vi "Sequence Execution.vi"() -> ()   [LabVIEW 2013, in "Simple Sequence Editor.lvlib"]
uses:
  Simple Sequence Editor.lvlib
  Types/Execute.PreviewMode.ctl
  Types/Execuction.StateVariables.ctl
  <vilib>/NI Veristand/Execution/Workspace/SystemStateRegEventRef.ctl
  <vilib>/NI Veristand/Execution/Workspace/SystemStateEventRef.ctl
  <vilib>/NI Veristand/Execution/Workspace/WorkspaceAPI.ctl
  Program Files/National Instruments/LabVIEW 2013/examples/NI Veristand/API/Execution API/Sequences/Stimulus Profile Control Tool/Project Execution State.ctl
  NationalInstruments.VeriStand.RealTimeSequenceDefinitionApi
  <vilib>/NI Veristand/Execution/Workspace/NI VeriStand - Get Single Channel Value.vi
  <vilib>/NI Veristand/Execution/Workspace/NI VeriStand - Set Single Channel Value.vi
  <vilib>/NI Veristand/Execution/Workspace/NI_VS Workspace ExecutionAPI.lvlib
  NationalInstruments.VeriStand.ClientAPI
panel:
  out "Current Step":u32
  out "Current Iteration":u32
  in  "NIVS.Project File Path":path
  in  "NIVS.Gateway IP Address":string="localhost"
  in  "NIVS.Workspace Event":refnum<event-registration>
  in  "Preview Mode":T1=enum."Table"
  in  "Start Step":u32 min=1 max=5
  in  "Start Iteration":u32=1 min=1 max=2
  in  "Log Channels":T2(ring)
  in  "Path":path
  in  "Enable Logging":bool
  in  "Abort":bool
  in  "Pause":bool
  in  "Start":bool
  in  "Profiles":string(combo)
  out "Graph":waveform(dbl)[](graph)
  out "Sequence":i32[](listbox)
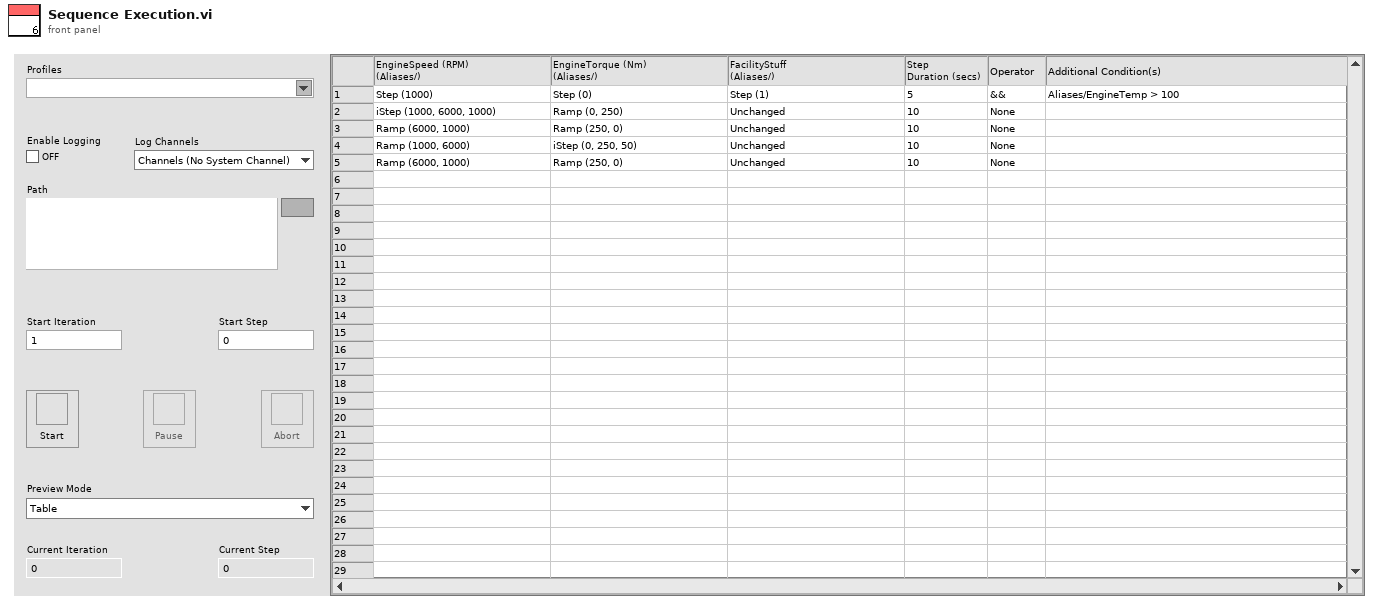
[diagram p1: front panel]
types:
  T1 = typedef "Simple Sequence Editor.lvlib/Execute.PreviewMode.ctl" = enum8{"Graph", "Table"}
  T2 = enum16{"Channels (No System Channel)", "Aliases", "All"}
  T3 = typedef "Simple Sequence Editor.lvlib/Execuction.StateVariables.ctl" = cluster{"Abort":refnum<vi>, "Pause":refnum<vi>, "Enable Logging":refnum<vi>, "Start":refnum<vi>, "Log Channels":refnum<vi>, "Start Iteration":refnum<vi>, "Start Step":refnum<vi>, "Sequence":refnum<vi>, "Preview Mode":refnum<vi>, "Graph":refnum<vi>, "Path":refnum<vi>, "NIVS.Events":cluster{"SequenceRef":refnum<event-registration>, "SystemChangeEventRef":T4, "NIVS.WorkspaceEvents":refnum<event-registration>}, "NIVS.SystemStateRefs":T5, "NIVS.WorkspaceManager":T6, "Abort 2":string, "Step":string, "Iterations":u32, "Iteration":string, "UI.Sequence#ofColumns":i32, "Connected":bool, "Profiles":refnum<vi>, "Events.State":refnum<user-event>, "Events.Test Result":refnum<user-event>, "Events.Progress":refnum<user-event>, "Profile.Ref":refnum<k24>, "Profile.Callback":refnum<k27>, "State":T7, "NIVS.Gateway IP Address":string, "NIVS.Project File Path":path, "Current Step":refnum<vi>, "Current Iteration":refnum<vi>}
  T4 = typedef "NI_VS Workspace ExecutionAPI.lvlib/SystemStateRegEventRef.ctl" = refnum<event-registration>
  T5 = typedef "NI_VS Workspace ExecutionAPI.lvlib/SystemStateEventRef.ctl" = cluster{"CustDatRef":refnum<user-event>, "EvtRef":refnum<k27>}
  T6 = typedef "NI_VS Workspace ExecutionAPI.lvlib/WorkspaceAPI.ctl" = refnum<k24>
  T7 = typedef "Project Execution State.ctl" = enum16{"Idle", "Initializing", "Running", "Paused", "Finalizing", "Complete"}
  T8 = cluster{"Event Registration Refnum":refnum<event-registration>, "SystemChangeEventRef":T4, "NIVS.Workspace Event":refnum<event-registration>}
  T9 = enum8{"Enabled", "Disabled", "Disabled and Grayed Out"}
  T10 = cluster{"SequenceRef":refnum<event-registration>, "SystemChangeEventRef":T4, "NIVS.WorkspaceEvents":refnum<event-registration>}
  T11 = typedef "NI_VS Workspace ExecutionAPI.lvlib/SystemState.ctl" = u8
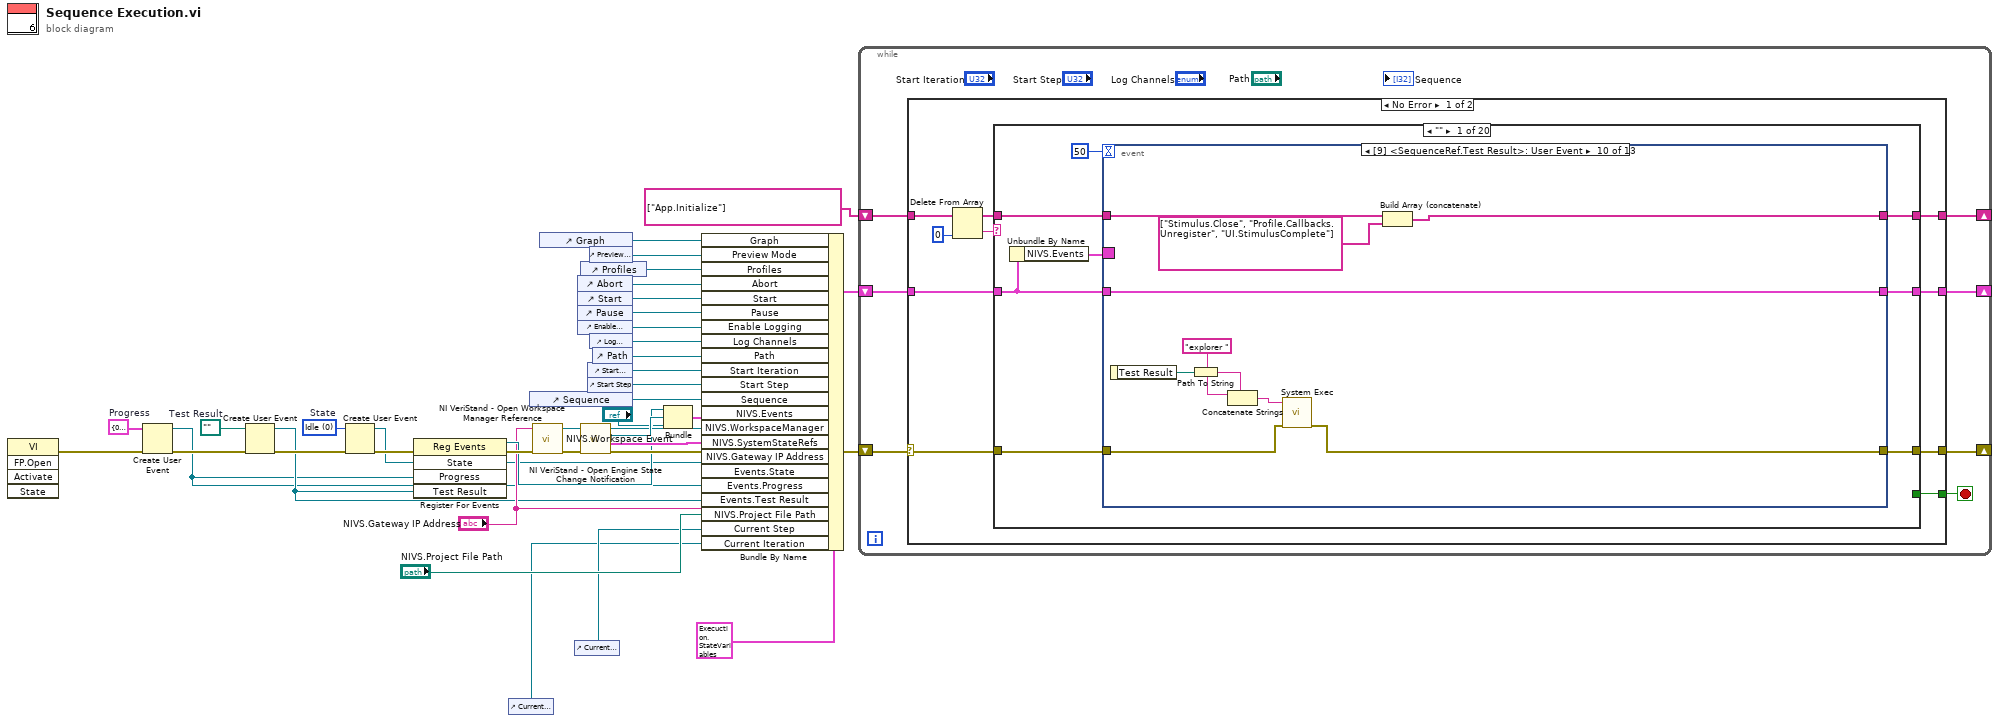
[diagram p0: block diagram]
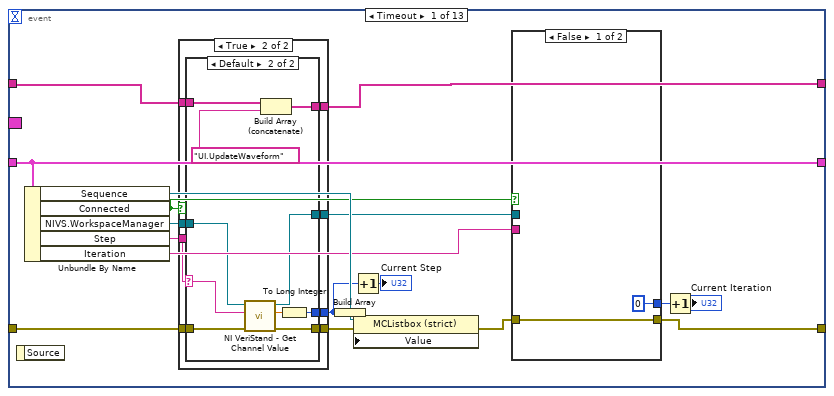
[diagram p2: hidden frame]
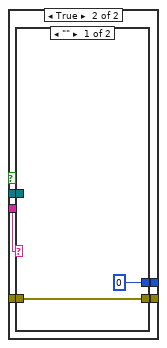
[diagram p3: hidden frame]
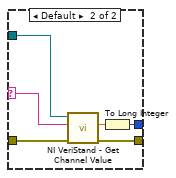
[diagram p4: hidden frame]
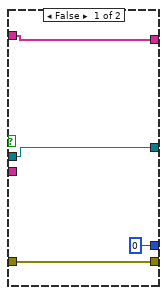
[diagram p5: hidden frame]
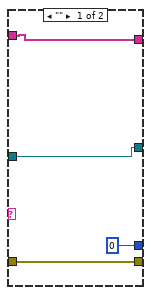
[diagram p6: hidden frame]
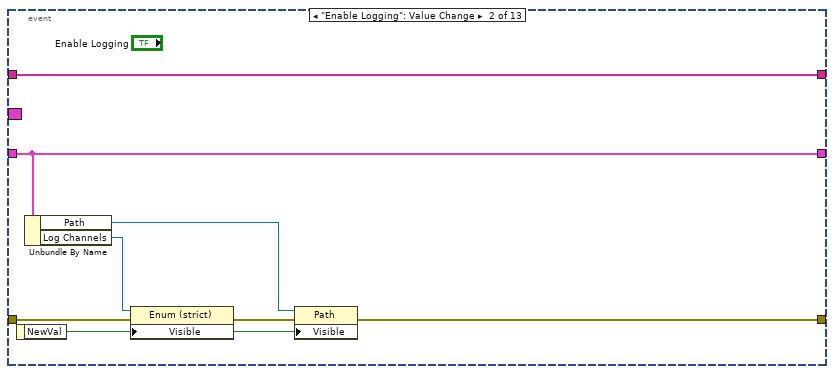
[diagram p7: hidden frame]
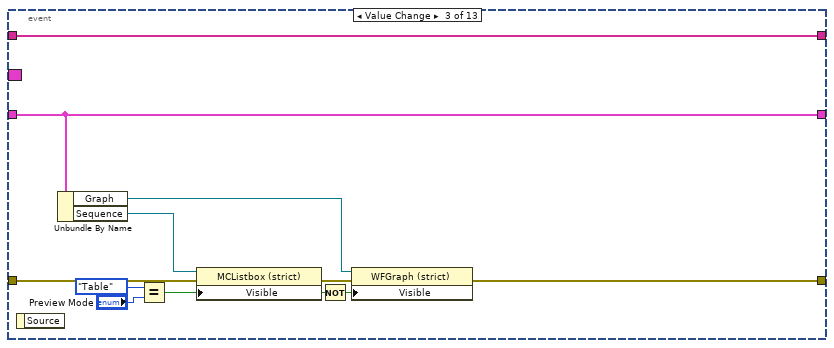
[diagram p8: hidden frame]
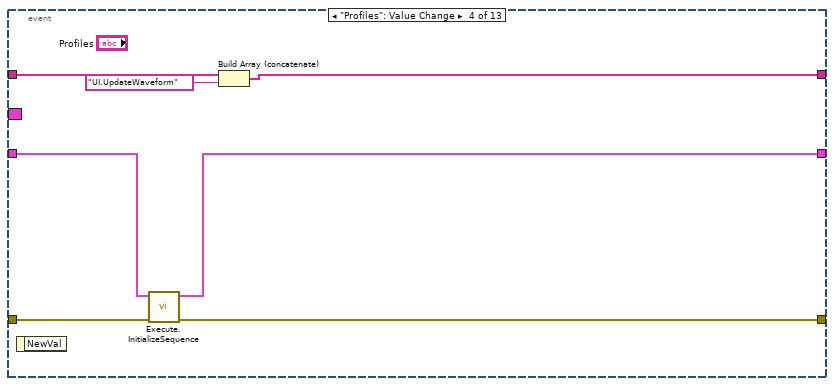
[diagram p9: hidden frame]
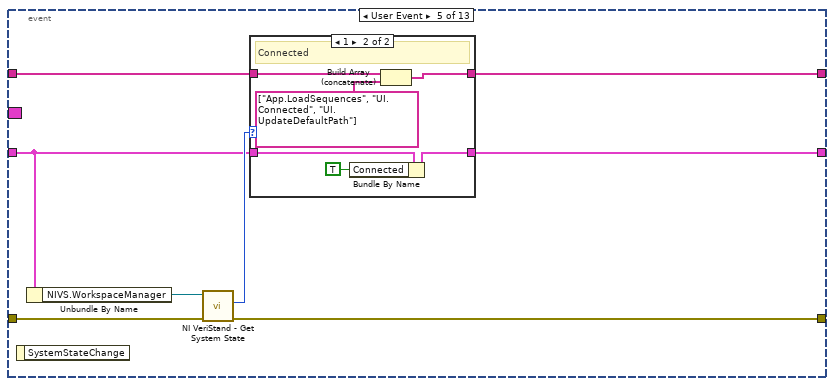
[diagram p10: hidden frame]
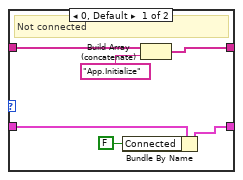
[diagram p11: hidden frame]
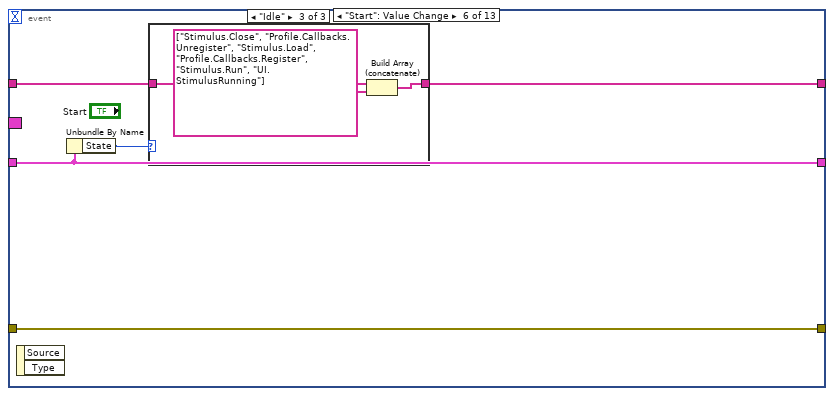
[diagram p12: hidden frame]
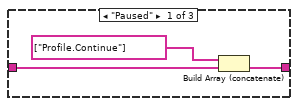
[diagram p13: hidden frame]
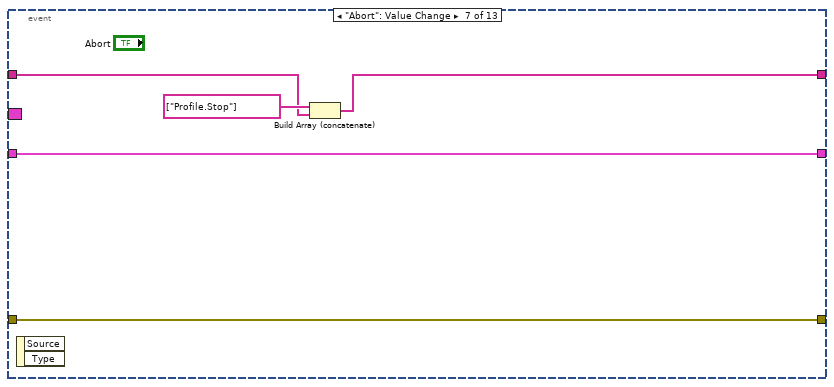
[diagram p15: hidden frame]
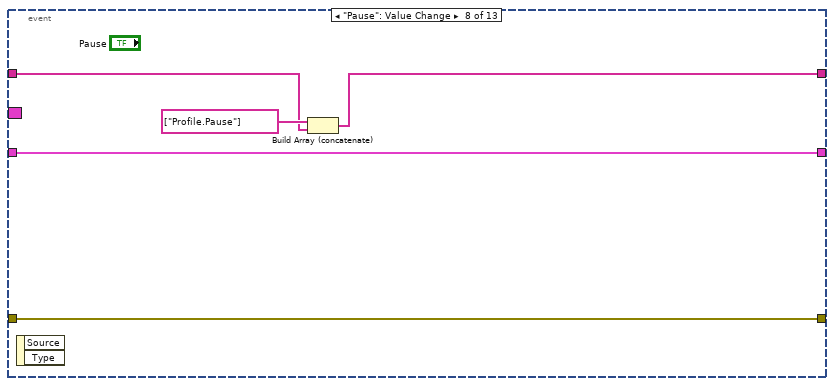
[diagram p16: hidden frame]
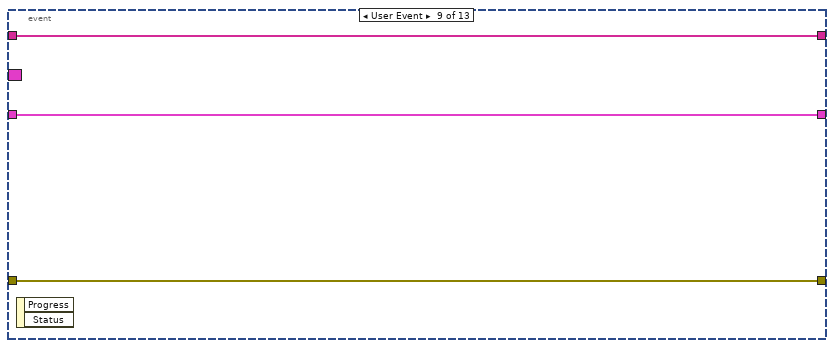
[diagram p17: hidden frame]
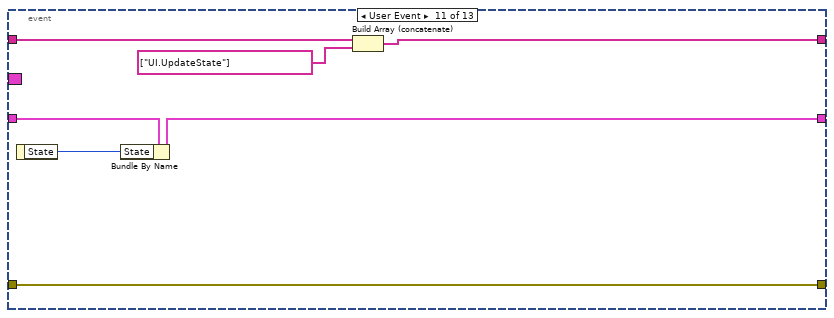
[diagram p18: hidden frame]
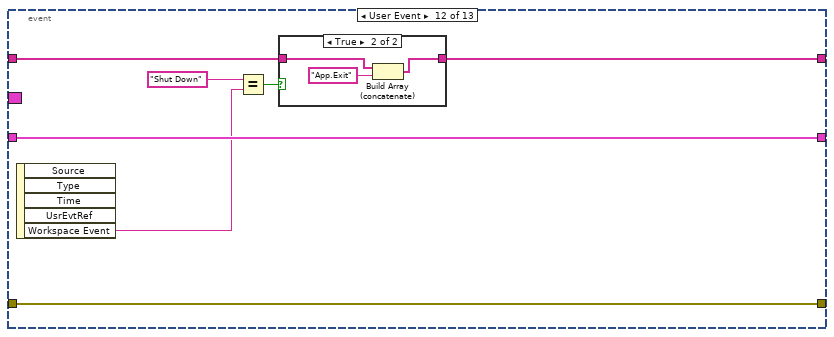
[diagram p19: hidden frame]
diagram:
  w11 = cluster{"Progress":dbl, "Status":string} {"Progress"=0.0, "Status"=""}  # Progress
  w17 = path ""  # Test Result
  w16 = 0 items=["Idle", "Initializing", "Running", "Paused", "Finalizing", "Complete"]  # State
  n1 = invoke class="VI" method="FP.Open"() -> (error out=w10:errorcluster)  [unwired: 5 in, 4 out]
  n2 = Create User Event(user event datatype=w11, error in=w10) -> (user event=w5:refnum<user-event>, error out=w9:errorcluster)
  n3 = Create User Event(user event datatype=w17, error in=w9) -> (user event=w6:refnum<user-event>, error out=w15:errorcluster)
  n4 = Create User Event(user event datatype=w16, error in=w15) -> (user event=w7:refnum<user-event>, error out=w14:errorcluster)
  n5 = register-events(error in=w14, w7, w5, w6) -> (reference out=w12:refnum<event-registration>, error out=w13:errorcluster)  [unwired: 1 in]
  n6 = control-ref of="Current Iteration"() -> (w1:refnum<vi>)
  n7 = control-ref of="Sequence"() -> (w23:refnum<vi>)
  n8 = call <vilib>:"NI VeriStand - Open Workspace Manager Reference.vi"("error in (no error)"=w13, "Gateway IP Address (\"\": localhost)"="NIVS.Gateway IP Address") -> ("error out"=w37:errorcluster, "WorkspaceManager"=w38:T6)  [unwired: 8 in]
  n9 = control-ref of="Graph"() -> (w33:refnum<vi>)
  n10 = control-ref of="Current Step"() -> (w2:refnum<vi>)
  n11 = control-ref of="Abort"() -> (w31:refnum<vi>)
  n12 = control-ref of="Start"() -> (w30:refnum<vi>)
  n13 = control-ref of="Pause"() -> (w29:refnum<vi>)
  n14 = control-ref of="Enable Logging"() -> (w28:refnum<vi>)
  n15 = control-ref of="Profiles"() -> (w19:refnum<vi>)
  n16 = call <vilib>:"NI VeriStand - Open Engine State Change Notification.vi"("error in (no error)"=w37, "WorkspaceManager in"=w38) -> ("error out"=w20:errorcluster, "SystemStateRefs"=w34:T5, "SystemChangeEventRef"=w36:T4, "WorkspaceManager out"=w22:T6)  [unwired: 6 in]
  n17 = control-ref of="Start Iteration"() -> (w25:refnum<vi>)
  n18 = control-ref of="Start Step"() -> (w24:refnum<vi>)
  n19 = control-ref of="Preview Mode"() -> (w32:refnum<vi>)
  n20 = control-ref of="Log Channels"() -> (w27:refnum<vi>)
  n21 = control-ref of="Path"() -> (w26:refnum<vi>)
  n22 = Bundle("Event Registration Refnum"=w12, "SystemChangeEventRef"=w36, "NIVS.Workspace Event"="NIVS.Workspace Event") -> (w35:T8)  [unwired: 1 in]
  n23 = Bundle By Name(cluster=T3 {"Abort"=refnum, "Pause"=refnum, "Enable Logging"=refnum, "Start"=refnum, "Log Channels"=refnum, "Start Iteration"=refnum, "Start Step"=refnum, "Sequence"=refnum, "Preview Mode"=refnum, "Graph"=refnum, "Path"=refnum, "NIVS.Events"={"SequenceRef"=refnum, "SystemChangeEventRef"=refnum, "NIVS.WorkspaceEvents"=refnum}, "NIVS.SystemStateRefs"={"CustDatRef"=refnum, "EvtRef"=refnum}, "NIVS.WorkspaceManager"=refnum, "Abort 2"="", "Step"="", "Iterations"=0, "Iteration"="", "UI.Sequence#ofColumns"=0, "Connected"=FALSE, "Profiles"=refnum, "Events.State"=refnum, "Events.Test Result"=refnum, "Events.Progress"=refnum, "Profile.Ref"=refnum, "Profile.Callback"=refnum, "State"=enum."Idle", "NIVS.Gateway IP Address"="", "NIVS.Project File Path"=path "", "Current Step"=refnum, "Current Iteration"=refnum} ("Cluster"), "Graph"=w33, "Preview Mode"=w32, "Profiles"=w19, "Abort"=w31, "Start"=w30, "Pause"=w29, "Enable Logging"=w28, "Log Channels"=w27, "Path"=w26, "Start Iteration"=w25, "Start Step"=w24, "Sequence"=w23, "NIVS.Events"=w35, "NIVS.WorkspaceManager"=w22, "NIVS.SystemStateRefs"=w34, "NIVS.Gateway IP Address"="NIVS.Gateway IP Address", "Events.State"=w7, "Events.Progress"=w5, "Events.Test Result"=w6, "NIVS.Project File Path"="NIVS.Project File Path", "Current Step"=w2, "Current Iteration"=w1) -> (w21:T3)
  n24 = while {
    shift-right: [w45] -> _
    shift-left: string[] ["App.Initialize"] -> [w46]
    shift-right: [w43] -> _
    shift-left: w21 -> [w44]
    shift-right: [w41] -> _
    shift-left: w20 -> [w42]
    stop <- w40 stop-if-true
    n25 = case shown="No Error" w42 {
      selector: w42 -> [w47 w418]
      tunnel: w46 -> [w49 w421]
      tunnel: [w55 w421] -> w45
      tunnel: w44 -> [w53 w420]
      tunnel: [w52 w420] -> w43
      tunnel: [w51 w417] -> w41
      tunnel: [w50 _] -> w40
      frame No Error {
        n26 = Delete From Array(array=w49, index=0) -> (deleted portion=w56:string, array with subset deleted=w54:string[])  [unwired: 1 in]
        n27 = case shown="\"\"" w56 {
          tunnel: [w62 w238 w242 w261 w266 w273 w274 w283 w293 w306 w335 w339 w342 w345 w354 w376 w380 w393 w413 w416] -> w55
          tunnel: w54 -> [w61 w238 w243 w261 w266 w273 w274 w283 w293 w306 w335 w339 w342 w345 w354 w376 w380 w393 w413 w416]
          tunnel: w53 -> [w58 w232 w240 w258 w263 w272 w276 w282 w292 w303 w324 w337 w340 w344 w348 w373 w377 w392 w406 w415]
          tunnel: [w64 w232 w239 w258 w262 w272 w276 w282 w292 w303 w323 w337 w340 w344 w348 w373 w377 w392 w406 w415] -> w52
          tunnel: [w59 w237 w244 w259 w264 w269 w277 w278 w288 w304 w330 w338 w341 w343 w352 w374 w378 w386 w403 w414] -> w51
          tunnel: w47 -> [w60 w237 w247 w260 w265 w270 w277 w279 w289 w305 w331 w338 w341 w343 w353 w375 w379 w389 w407 w414]
          tunnel: [_ TRUE _ _ _ _ _ _ _ _ _ _ _ _ _ _ _ _ _ _] -> w50
          frame "" {
            n28 = Unbundle By Name(w58) -> ("NIVS.Events"=w57:T10)
            n29 = event shown="[9] <SequenceRef.Test Result>: User Event" {
              selector: w57 -> [_ _ _ _ _ _ _ _ _ _ _ _ _]
              dyn-events: _ -> [_ _ _ _ _ _ _ _ _ _ _ _ _]
              timeout: 50 -> [_ _ _ _ _ _ _ _ _ _ _ _ _]
              tunnel: [w74 w131 w142 w143 w152 w172 w182 w187 w194 w202 w205 w213 w224] -> w62
              tunnel: w61 -> [w75 w131 w142 w144 w153 w173 w183 w188 w194 w203 w206 w216 w228]
              tunnel: [w82 w130 w139 w146 w150 w171 w186 w191 w193 w204 w208 w218 w227] -> w64
              tunnel: w58 -> [w82 w130 w139 w147 w151 w171 w186 w191 w193 w204 w209 w218 w227]
              tunnel: [w65 w124 w132 w148 w154 w174 w185 w190 w192 w199 w211 w217 w226] -> w59
              tunnel: w60 -> [w80 w128 w133 w149 w155 w174 w185 w190 w192 w200 w211 w217 w226]
              event Timeout {
                n30 = event-data() -> ()  [unwired: 1 in, 1 out]
                n31 = Unbundle By Name(w82) -> ("Sequence"=w78:refnum<vi>, "Connected"=w73:bool, "NIVS.WorkspaceManager"=w81:T6, "Step"=w79:string, "Iteration"=w71:string)
                n32 = case shown="True" w73 {
                  tunnel: w81 -> [w98 w107]
                  tunnel: w80 -> [w101 w109]
                  tunnel: [w101 w108] -> w77
                  tunnel: w79 -> [_ w105]
                  tunnel: [0 w106] -> w70
                  tunnel: w75 -> [w99 w104]
                  tunnel: [w99 w103] -> w74
                  tunnel: [w98 w102] -> w72
                  frame False {
                  }
                  frame True {
                    n33 = case shown="Default" w105 {
                      selector: w105 -> [_ w118]
                      tunnel: w109 -> [w113 w123]
                      tunnel: [w113 w122] -> w108
                      tunnel: w107 -> [w110 w121]
                      tunnel: [0 w119] -> w106
                      tunnel: w104 -> [w111 w116]
                      tunnel: [w111 w115] -> w103
                      tunnel: [w110 w114] -> w102
                      frame "" {
                      }
                      frame Default {
                        n34 = call-poly <vilib>:"NI VeriStand - Get Channel Value.vi"("error in (no error)"=w123, "Channel"=w118, "WorkspaceManager in"=w121) -> ("error out"=w122:errorcluster, "Value"=w120:dbl, "WorkspaceManager out"=w114:T6)  [unwired: 6 in]
                        n35 = Build Array (concatenate)(w116, "UI.UpdateWaveform") -> (w115:string[])
                        n36 = To Long Integer(number=w120) -> (32bit integer=w119:i32)
                      }
                    }
                  }
                }
                n37 = Build Array(w70) -> (w76:i32[])
                n38 = Increment(x=w70) -> (x+1=→"Current Step":i32)
                n39 = property class="MCListbox (strict)"(reference=w78, error in=w77, "Value"=w76) -> (error out=w66:errorcluster)  [unwired: 1 out]
                n40 = case shown="False" w73 {
                  tunnel: w72 -> [_ w87]
                  tunnel: w66 -> [w84 w89]
                  tunnel: [w84 w88] -> w65
                  tunnel: w71 -> [_ w85]
                  tunnel: [0 w86] -> w68
                  frame False {
                  }
                  frame True {
                    n41 = case shown="\"\"" w85 {
                      selector: w85 -> [_ w92]
                      tunnel: w89 -> [w91 w97]
                      tunnel: [w91 w96] -> w88
                      tunnel: w87 -> [_ w95]
                      tunnel: [0 w93] -> w86
                      frame "" {
                      }
                      frame Default {
                        n42 = call-poly <vilib>:"NI VeriStand - Get Channel Value.vi"("error in (no error)"=w97, "Channel"=w92, "WorkspaceManager in"=w95) -> ("error out"=w96:errorcluster, "Value"=w94:dbl)  [unwired: 6 in, 1 out]
                        n43 = To Long Integer(number=w94) -> (32bit integer=w93:i32)
                      }
                    }
                  }
                }
                n44 = Increment(x=w68) -> (x+1=→"Current Iteration":i32)
              }
              event "Enable Logging": Value Change {
                n45 = event-data() -> ("NewVal"=w125:bool)  [unwired: 1 in]
                n46 = Unbundle By Name(w130) -> ("Path"=w126:refnum<vi>, "Log Channels"=w129:refnum<vi>)
                n47 = property class="Enum (strict)"(reference=w129, error in=w128, "Visible"=w125) -> (error out=w127:errorcluster)  [unwired: 1 out]
                n48 = property class="Path"(reference=w126, error in=w127, "Visible"=w125) -> (error out=w124:errorcluster)  [unwired: 1 out]
              }
              event Value Change {
                n49 = event-data() -> ()  [unwired: 1 in, 1 out]
                n50 = Unbundle By Name(w139) -> ("Graph"=w137:refnum<vi>, "Sequence"=w138:refnum<vi>)
                n51 = Equal?(x=Execute.PreviewMode."Table" ("y"), y="Preview Mode") -> (x = y?=w135:bool)
                n52 = property class="MCListbox (strict)"(reference=w138, error in=w133, "Visible"=w135) -> (error out=w136:errorcluster)  [unwired: 1 out]
                n53 = Not(x=w135) -> (.not. x?=w134:bool)
                n54 = property class="WFGraph (strict)"(reference=w137, error in=w136, "Visible"=w134) -> (error out=w132:errorcluster)  [unwired: 1 out]
              }
              event "Profiles": Value Change {
                n55 = event-data() -> ()  [unwired: 1 in, 1 out]
                n56 = call "Execute.InitializeSequence.vi"("error in (no error)"=w149, "State Variables"=w147) -> ("error out"=w148:errorcluster, "State Variables"=w146:T3)  [unwired: 8 in]
                n57 = Build Array (concatenate)(w144, "UI.UpdateWaveform") -> (w143:string[])
              }
              event User Event {
                n58 = event-data() -> ()  [unwired: 1 in, 1 out]
                n59 = Unbundle By Name(w151) -> ("NIVS.WorkspaceManager"=w157:T6)
                n60 = call <vilib>:"NI VeriStand - Get System State.vi"("error in (no error)"=w155, "WorkspaceManager in"=w157) -> ("error out"=w154:errorcluster, "System State"=w156:T11)  [unwired: 5 in, 3 out]
                n61 = case shown="1" w156 {
                  tunnel: w153 -> [w163 w169]
                  tunnel: [w162 w168] -> w152
                  tunnel: w151 -> [w159 w166]
                  tunnel: [w158 w165] -> w150
                  frame 0, Default {
                    # "Not connected"
                    n62 = Bundle By Name(cluster=w159, "Connected"=FALSE) -> (w158:T3)
                    n63 = Build Array (concatenate)(w163, "App.Initialize") -> (w162:string[])
                  }
                  frame 1 {
                    # "Connected"
                    n64 = Bundle By Name(cluster=w166, "Connected"=TRUE) -> (w165:T3)
                    n65 = Build Array (concatenate)(w169, string[] ["App.LoadSequences", "UI.Connected", "UI.UpdateDefaultPath"]) -> (w168:string[])
                  }
                }
              }
              event "Start": Value Change {
                n66 = event-data() -> ()  [unwired: 1 in, 2 out]
                n67 = Unbundle By Name(w171) -> ("State"=w170:T7)
                n68 = case shown="\"Idle\"" w170 {
                  tunnel: w173 -> [w176 w178 w181]
                  tunnel: [w175 w178 w180] -> w172
                  frame "Paused" {
                    n69 = Build Array (concatenate)(string[] ["Profile.Continue"] ("array"), w176) -> (w175:string[])
                  }
                  frame Default {
                  }
                  frame "Idle" {
                    n70 = Build Array (concatenate)(w181, string[] ["Stimulus.Close", "Profile.Callbacks.Unregister", "Stimulus.Load", "Profile.Callbacks.Register", "Stimulus.Run", "UI.StimulusRunning"] ("array")) -> (w180:string[])
                  }
                }
              }
              event "Abort": Value Change {
                n71 = event-data() -> ()  [unwired: 1 in, 2 out]
                n72 = Build Array (concatenate)(string[] ["Profile.Stop"] ("array"), w183) -> (w182:string[])
              }
              event "Pause": Value Change {
                n73 = event-data() -> ()  [unwired: 1 in, 2 out]
                n74 = Build Array (concatenate)(string[] ["Profile.Pause"] ("array"), w188) -> (w187:string[])
              }
              event User Event {
                n75 = event-data() -> ()  [unwired: 1 in, 2 out]
              }
              event User Event {
                n76 = event-data() -> ("Test Result"=w198:path)  [unwired: 1 in]
                n77 = Path To String(path=w198) -> (string=w197:string)
                n78 = Concatenate Strings("explorer " ("string"), w197) -> (w196:string)
                n79 = call <vilib>:"System Exec.vi"("error in (no error)"=w200, "command line"=w196) -> ("error out"=w199:errorcluster)  [unwired: 6 in, 3 out]
                n80 = Build Array (concatenate)(w203, string[] ["Stimulus.Close", "Profile.Callbacks.Unregister", "UI.StimulusComplete"]) -> (w202:string[])
              }
              event User Event {
                n81 = event-data() -> ("State"=w210:i32)  [unwired: 1 in]
                n82 = Bundle By Name(cluster=w209, "State"=w210) -> (w208:T3)
                n83 = Build Array (concatenate)(w206, string[] ["UI.UpdateState"] ("array")) -> (w205:string[])
              }
              event User Event {
                n84 = event-data() -> ("Workspace Event"=w212:string)  [unwired: 1 in, 4 out]
                n85 = Equal?(x="Shut Down" ("y"), y=w212) -> (x = y?=w214:bool)
                n86 = case shown="True" w214 {
                  tunnel: w216 -> [w219 w222]
                  tunnel: [w219 w220] -> w213
                  frame False {
                  }
                  frame True {
                    n87 = Build Array (concatenate)(w222, "App.Exit" ("y")) -> (w220:string[])
                  }
                }
              }
              event Panel Close? {
                n88 = event-data() -> ()  [unwired: 1 in, 1 out]
                n89 = Build Array (concatenate)(w228, "App.Exit") -> (w224:string[])
                n90 = event-data("Discard?"=TRUE) -> ()  [unwired: 1 in, 1 out]
              }
            }
          }
          frame "App.Exit" {
            n91 = Unbundle By Name(w232) -> ("Events.State"=w233:refnum<user-event>, "Events.Test Result"=w234:refnum<user-event>, "Events.Progress"=w235:refnum<user-event>, "NIVS.Events"=w231:T10, "NIVS.SystemStateRefs"=w230:T5, "NIVS.WorkspaceManager"=w229:T6)
            n92 = call <vilib>:"NI VeriStand - Close Workspace Manager Reference.vi"("WorkspaceManager"=w229) -> ()  [unwired: 10 in, 1 out]
            n93 = call <vilib>:"NI VeriStand - Close Engine State Change Notification.vi"("SystemStateRefs"=w230) -> ()  [unwired: 10 in, 1 out]
            n94 = Unregister For Events(event registration refnum=w231) -> ()  [unwired: 1 in, 1 out]
            n95 = Destroy User Event(user event=w235) -> ()  [unwired: 1 in, 1 out]
            n96 = Destroy User Event(user event=w234) -> ()  [unwired: 1 in, 1 out]
            n97 = Destroy User Event(user event=w233) -> ()  [unwired: 1 in, 1 out]
            n98 = invoke class="VI" method="FP.Close"() -> ()  [unwired: 3 in, 3 out]
          }
          frame "App.Initialize" {
            n99 = Unbundle By Name(w240) -> ("NIVS.WorkspaceManager"=w241:T6)
            n100 = call "Execute.Initialize.vi"("error in (no error)"=w247, "Cluster"=w240) -> ("error out"=w245:errorcluster)  [unwired: 9 in]
            n101 = call <vilib>:"NI VeriStand - Get System State.vi"("error in (no error)"=w245, "WorkspaceManager in"=w241) -> ("error out"=w244:errorcluster, "System State"=w246:T11)  [unwired: 5 in, 3 out]
            n102 = case shown="1" w246 {
              tunnel: w243 -> [w251 w257]
              tunnel: [w251 w256] -> w242
              tunnel: w240 -> [w250 w254]
              tunnel: [w249 w252] -> w239
              frame 0, Default {
                # "Not connected"
                n103 = Bundle By Name(cluster=w250, "Connected"=FALSE) -> (w249:T3)
              }
              frame 1 {
                # "Connected"
                n104 = Bundle By Name(cluster=w254, "Connected"=TRUE) -> (w252:T3)
                n105 = Build Array (concatenate)(w257, string[] ["App.LoadSequences", "UI.Connected", "UI.UpdateDefaultPath"]) -> (w256:string[])
              }
            }
          }
          frame "App.LoadSequences" {
            n106 = call "Execute.LoadSequences.vi"("error in (no error)"=w260, "Cluster"=w258) -> ("error out"=w259:errorcluster)  [unwired: 9 in]
          }
          frame "Stimulus.Load" {
            n107 = call "Execute.RunStimulus.vi"("error in (no error)"=w265, "State Variables"=w263) -> ("error out"=w264:errorcluster, "State Variables"=w262:T3)  [unwired: 8 in]
          }
          frame "Stimulus.Run" {
            n108 = Unbundle By Name(w272) -> ("Profile.Ref"=w271:refnum<k24>, "NIVS.Gateway IP Address"=w267:string)
            n109 = invoke class="StimulusProfile" method="ExecuteAsync"(reference=w271, error in=w270, "gatewayIP"=w267, "uutSerialNumber"="") -> (error out=w269:errorcluster)  [unwired: 1 in, 4 out]
          }
          frame "Stimulus.Close" {
            n110 = Unbundle By Name(w276) -> ("Profile.Ref"=w275:refnum<k24>)
            n111 = Close Reference(reference=w275) -> ()  [unwired: 1 in, 1 out]
          }
          frame "Profile.Pause" {
            n112 = Unbundle By Name(w282) -> ("State"=w280:T7, "Profile.Ref"=w281:refnum<k24>)
            n113 = case shown="\"Running\"" w280 {
              tunnel: w281 -> [_ w287]
              tunnel: w279 -> [w284 w286]
              tunnel: [w284 w285] -> w278
              frame "Idle", Default {
              }
              frame "Running" {
                n114 = invoke class="StimulusProfile" method="Pause"(reference=w287, error in=w286) -> (error out=w285:errorcluster)  [unwired: 1 in, 2 out]
              }
            }
          }
          frame "Profile.Continue" {
            n115 = Unbundle By Name(w292) -> ("State"=w291:T7, "Profile.Ref"=w290:refnum<k24>)
            n116 = case shown="\"Paused\"" w291 {
              tunnel: w290 -> [_ w297]
              tunnel: w289 -> [w294 w296]
              tunnel: [w294 w295] -> w288
              frame "Idle", Default {
              }
              frame "Paused" {
                n117 = invoke class="StimulusProfile" method="Continue"(reference=w297, error in=w296) -> (error out=w295:errorcluster)  [unwired: 1 in, 2 out]
              }
            }
          }
          frame "Profile.Stop" {
            n118 = Unbundle By Name(w303) -> ("Sequence"=w298:refnum<vi>, "NIVS.WorkspaceManager"=w299:T6, "Abort 2"=w300:string, "State"=w301:T7, "Profile.Ref"=w302:refnum<k24>)
            n119 = case shown="\"Running\", \"Paused\", Default" w301 {
              tunnel: w302 -> [_ w312]
              tunnel: w305 -> [w307 w316]
              tunnel: [w307 w309] -> w304
              tunnel: w300 -> [_ w315]
              tunnel: w299 -> [_ w314]
              tunnel: w298 -> [_ w311]
              frame "Idle" {
              }
              frame "Running", "Paused", Default {
                n120 = case shown="Default" w315 {
                  selector: w315 -> [_ w319]
                  tunnel: w316 -> [w317 w322]
                  tunnel: [w317 w321] -> w313
                  tunnel: w314 -> [_ w320]
                  frame "" {
                  }
                  frame Default {
                    n121 = call-poly <vilib>:"NI VeriStand - Set Channel Value.vi"("error in (no error)"=w322, "Value"=1.0, "Channel"=w319, "WorkspaceManager in"=w320) -> ("error out"=w321:errorcluster)  [unwired: 6 in, 1 out]
                  }
                }
                n122 = invoke class="StimulusProfile" method="Stop"(reference=w312, error in=w313) -> (error out=w310:errorcluster)  [unwired: 1 in, 2 out]
                n123 = property class="MCListbox (strict)"(reference=w311, error in=w310, "Value"=i32[] [0]) -> (error out=w309:errorcluster)  [unwired: 1 out]
              }
            }
          }
          frame "Profile.Callbacks.Register" {
            n124 = Unbundle By Name(w324) -> ("Profile.Ref"=w329:refnum<k24>, "Events.Progress"=w328:refnum<user-event>, "Events.Test Result"=w327:refnum<user-event>, "Events.State"=w326:refnum<user-event>)
            n125 = vi-ref "PropertyChanged Event Callback.vi"() -> ("vi reference"=w332:refnum<vi>)
            n126 = vi-ref "ProgressChanged Event Callback.vi"() -> ("vi reference"=w334:refnum<vi>)
            n127 = vi-ref "ExecuteCompleted Event Callback.vi"() -> ("vi reference"=w333:refnum<vi>)
            n128 = node(w331, w329, w334, w328, w329, w333, w327, w329, w332, w326) -> (w325:refnum<k27>, w330:errorcluster)  [unwired: 1 in]
            n129 = Bundle By Name(cluster=w324, "Profile.Callback"=w325) -> (w323:T3)
          }
          frame "Profile.Callbacks.Unregister" {
            n130 = Unbundle By Name(w337) -> ("Profile.Callback"=w336:refnum<k27>)
            n131 = Unregister For Events(event registration refnum=w336) -> ()  [unwired: 1 in, 1 out]
          }
          frame "Sequence.Build" {
          }
          frame "Sequence.Validate" {
          }
          frame "UI.UpdateWaveform" {
            n132 = Unbundle By Name(w348) -> ("State"=w347:T7, "Graph"=w349:refnum<vi>, "Sequence"=w350:refnum<vi>, "UI.Sequence#ofColumns"=w351:i32)
            n133 = case shown="Default" w347 {
              tunnel: w353 -> [w361 w367]
              tunnel: [w360 w372] -> w352
              tunnel: w351 -> [w358 w370]
              tunnel: w350 -> [w357 w365]
              tunnel: w349 -> [w356 w369]
              tunnel: [w355 w368] -> w346
              frame "Idle" {
                n134 = call "Sequence.BuildPreviewWaveform.vi"("WaveformGraph in"=w356, "error in (no error)"=w361, "Rows"=cluster{"Start Index":i32, "Length":i32} {"Start Index"=0, "Length"=-1}, "UI.Sequence#ofColumns"=w358, "SequenceRef"=w357) -> ("error out"=w360:errorcluster, "Wavefrom"=w355:waveform(dbl)[])  [unwired: 5 in]
              }
              frame Default {
                n135 = property class="MCListbox (strict)"(reference=w365, error in=w367) -> (error out=w366:errorcluster, "Value"=w363:i32[])  [unwired: 1 out]
                n136 = Index Array(array=w363) -> (element=w362:i32)  [unwired: 1 in]
                n137 = Bundle By Name(cluster=cluster{"Start Index":i32, "Length":i32} {"Start Index"=0, "Length"=1} ("Rows"), "Start Index"=w362) -> (w364:cluster{"Start Index":i32, "Length":i32})
                n138 = call "Sequence.BuildPreviewWaveform.vi"("WaveformGraph in"=w369, "error in (no error)"=w366, "Rows"=w364, "UI.Sequence#ofColumns"=w370, "SequenceRef"=w365) -> ("error out"=w372:errorcluster, "Wavefrom"=w368:waveform(dbl)[])  [unwired: 5 in]
              }
            }
            "Graph" <- w346
          }
          frame "UI.StimulusRunning" {
            n139 = call "Execute.UI.Running.vi"("error in (no error)"=w375, "Cluster"=w373) -> ("error out"=w374:errorcluster)  [unwired: 9 in]
          }
          frame "UI.StimulusComplete" {
            n140 = call "Execute.UI.Complete.vi"("error in (no error)"=w379, "Cluster"=w377) -> ("error out"=w378:errorcluster)  [unwired: 9 in]
          }
          frame "UI.UpdateState" {
            n141 = Unbundle By Name(w392) -> ("Start"=w382:refnum<vi>, "Abort"=w383:refnum<vi>, "Pause"=w390:refnum<vi>, "State"=w391:T7)
            n142 = case shown="\"Running\"" w391 {
              tunnel: [w395 w396 T9."Disabled and Grayed Out" ("Disabled") w400] -> w385
              tunnel: [T9."Disabled and Grayed Out" ("Disabled") w396 w397 T9."Enabled" ("f")] -> w381
              tunnel: [w395 w396 w397 w400] -> w384
              frame "Running" {
                w395 = T9."Enabled" ("Disabled")
              }
              frame Default {
                w396 = T9."Disabled and Grayed Out" ("Disabled")
              }
              frame "Paused" {
                w397 = T9."Enabled" ("Disabled")
              }
              frame "Idle" {
                w400 = T9."Disabled and Grayed Out" ("Disabled")
              }
            }
            n143 = property class="Bool"(reference=w390, error in=w389, "DisabledEnum"=w385) -> (error out=w388:errorcluster)  [unwired: 1 out]
            n144 = property class="Bool"(reference=w383, error in=w388, "DisabledEnum"=w384) -> (error out=w387:errorcluster)  [unwired: 1 out]
            n145 = property class="Bool"(reference=w382, error in=w387, "DisabledEnum"=w381) -> (error out=w386:errorcluster)  [unwired: 1 out]
          }
          frame "UI.UpdateDefaultPath" {
            n146 = Unbundle By Name(w406) -> ("Path"=w402:refnum<vi>, "NIVS.WorkspaceManager"=w405:T6)
            n147 = call <vilib>:"NI VeriStand - Get System State.vi"("error in (no error)"=w407, "WorkspaceManager in"=w405) -> ("error out"=w404:errorcluster, "System Definition File"=w408:path)  [unwired: 5 in, 3 out]
            n148 = Strip Path(path=w408) -> (stripped path=w412:path)  [unwired: 1 out]
            n149 = Build Path(base path=path "Logs" ("stripped path"), name or relative path="Log.TDMS") -> (appended path=w410:path)
            n150 = Build Path(base path=w412, name or relative path=w410) -> (appended path=w401:path)
            n151 = property class="Path"(reference=w402, error in=w404, "Value"=w401) -> (error out=w403:errorcluster)  [unwired: 1 out]
          }
          frame Default {
          }
        }
      }
      frame Error {
        n152 = call <vilib>:"Simple Error Handler.vi"("error in (no error)"=w418) -> ("error out"=w419:errorcluster)  [unwired: 4 in, 4 out]
        n153 = call <vilib>:"Clear Errors.vi"("error in (no error)"=w419) -> ("error out"=w417:errorcluster)  [unwired: 6 in]
      }
    }
  }
